vi "DataGraph_MouseUp.vi"(8 "error in (no error)":errorcluster, 11 "Mass_Graph":refnum<vi>) -> (0 "error out":errorcluster, 2 "Rectangle Y":cluster{"Minimum":dbl, "Maximum":dbl}, 3 "Rectangle X":cluster{"Minimum":dbl, "Maximum":dbl}, 5 "Allow Index Bool":bool[](array[boolean]))   [LabVIEW 2018, in "DataGraphXControl.xctl"]
uses:
  DataGraphXControl.xctl
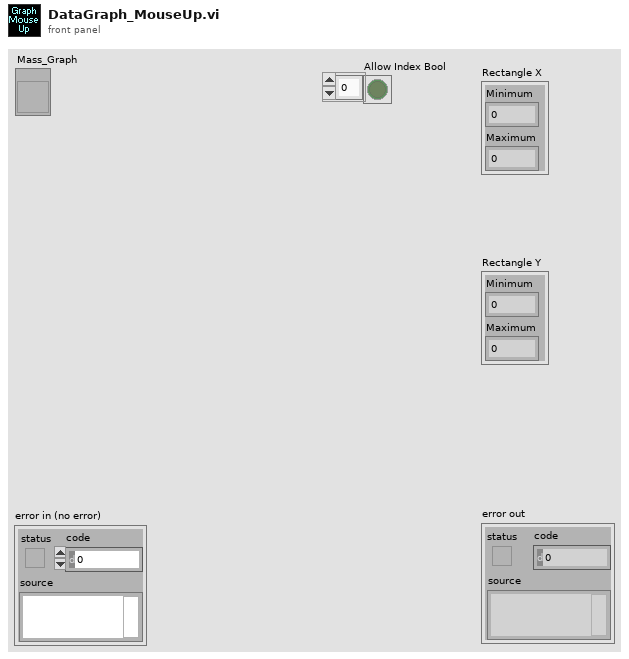
[diagram p1: front panel]
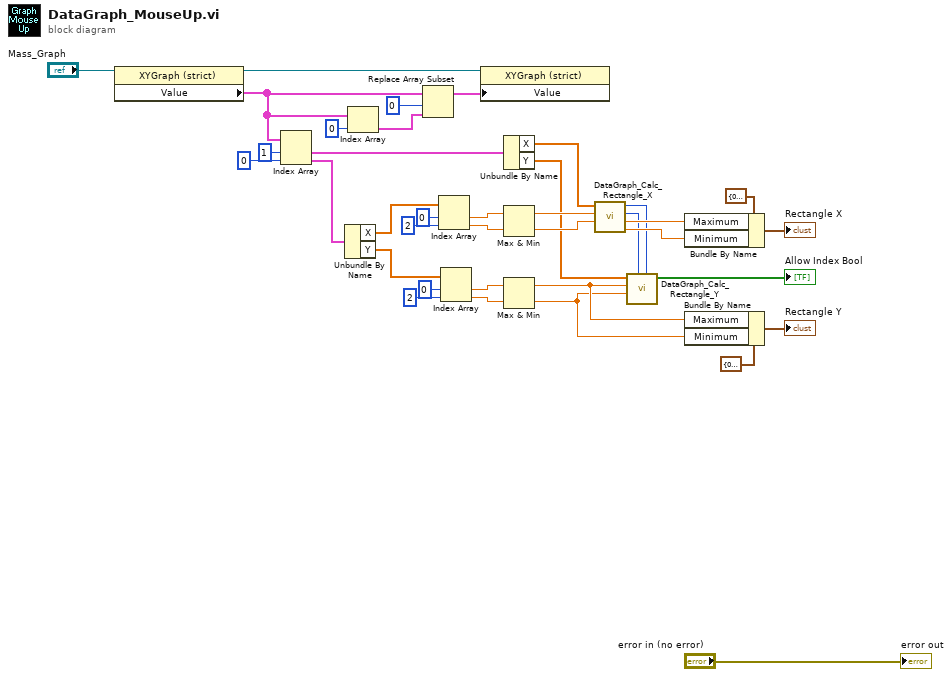
[diagram p0: block diagram]
diagram:
  n1 = property class="XYGraph (strict)"(reference="Mass_Graph") -> (reference out=w35:refnum<vi>, "Value"=w11:cluster{"X":dbl[], "Y":dbl[]}[])  [unwired: 1 in, 1 out]
  n2 = Index Array(array=w11, index #1=1 ("index"), index #2=0 ("index")) -> (element #1=w21:cluster{"X":dbl[], "Y":dbl[]}, element #2=w22:cluster{"X":dbl[], "Y":dbl[]})
  n3 = Unbundle By Name(w22) -> ("X"=w34:dbl[], "Y"=w25:dbl[])
  n4 = Index Array(array=w11, index=0) -> (element=w8:cluster{"X":dbl[], "Y":dbl[]})
  n5 = Replace Array Subset(array=w11, new element=w8, index=0) -> (w10:cluster{"X":dbl[], "Y":dbl[]}[])
  n6 = Index Array(array=w34, index #1=0 ("index"), index #2=2 ("index")) -> (element #1=w31:dbl, element #2=w30:dbl)
  n7 = Index Array(array=w25, index #1=0 ("index"), index #2=2 ("index")) -> (element #1=w27:dbl, element #2=w26:dbl)
  n8 = property class="XYGraph (strict)"(reference=w35, "Value"=w10) -> ()  [unwired: 1 in, 2 out]
  n9 = Unbundle By Name(w21) -> ("X"=w6:dbl[], "Y"=w5:dbl[])
  n10 = Max & Min(x=w31, y=w30) -> (max(x,y)=w19:dbl, min(x,y)=w20:dbl)
  n11 = Max & Min(x=w27, y=w26) -> (max(x,y)=w2:dbl, min(x,y)=w1:dbl)
  n12 = call "DataGraph_Calc_Rectangle_X.vi"("Minimum X"=w20, "Maximum X"=w19, "Raw X Array"=w6) -> ("Minimum Value"=w16:dbl, "Maximum Value"=w17:dbl, "Minimum Index"=w4:u32, "Maximum Index"=w3:u32)  [unwired: 5 in]
  n13 = call "DataGraph_Calc_Rectangle_Y.vi"("X Maximum Index"=w3, "X Minimum Index"=w4, "Y Minimum"=w1, "Y Maximum"=w2, "Raw Y Array"=w5) -> ("Allow Index Bool"=→"Allow Index Bool":bool[])  [unwired: 4 in]
  n14 = Bundle By Name(cluster=cluster{"Minimum":dbl, "Maximum":dbl} {"Minimum"=0.0, "Maximum"=0.0} ("Rectangle X"), "Maximum"=w17, "Minimum"=w16) -> (→"Rectangle X":cluster{"Minimum":dbl, "Maximum":dbl})
  n15 = Bundle By Name(cluster=cluster{"Minimum":dbl, "Maximum":dbl} {"Minimum"=0.0, "Maximum"=0.0} ("Rectangle Y"), "Maximum"=w2, "Minimum"=w1) -> (→"Rectangle Y":cluster{"Minimum":dbl, "Maximum":dbl})
  "error out" <- "error in (no error)"
